vi "Host Input to FPGA_5772_Sine.vi"() -> ()   [LabVIEW 2011]
panel:
  in  "millisecond multiple":u32=20
  out "Trig Offset":u8
  out "16bit integer":i16[](array[numeric])
  out "Init Data":i16[](array[numeric])
  in  "Marker Position":u32
  in  "Frequency":dbl=10000000.0 format="%#_p"
  in  "signal type":T1(ring)
  in  "stop":bool
  out "Data Generated":cluster{"Data":i16, i16}(graph)
  in  "sampling info":cluster{"Fs":dbl, "#s":dbl}={"Fs"=250000000.0, "#s"=100.0} {"Fs" format="%#_p"}
  # "You cannot change waveform type on the fly"
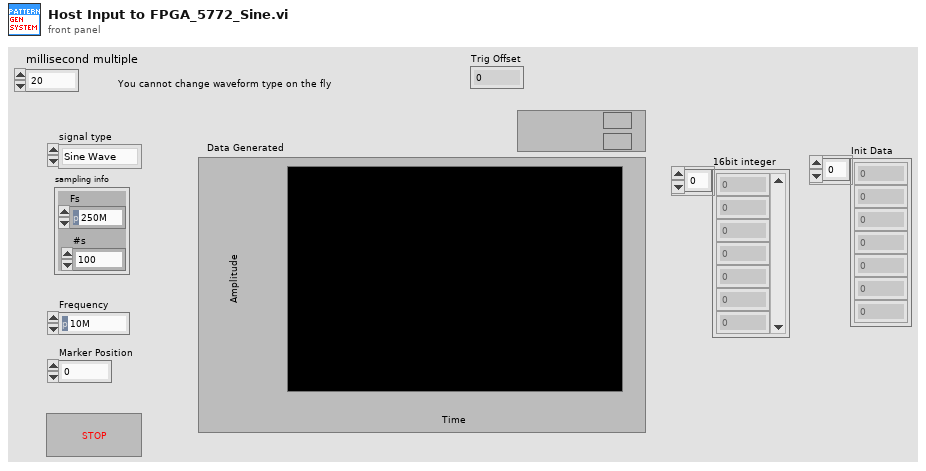
[diagram p1: front panel]
types:
  T1 = enum16{"Sine Wave", "Triangle Wave", "Square Wave", "Sawtooth Wave"}
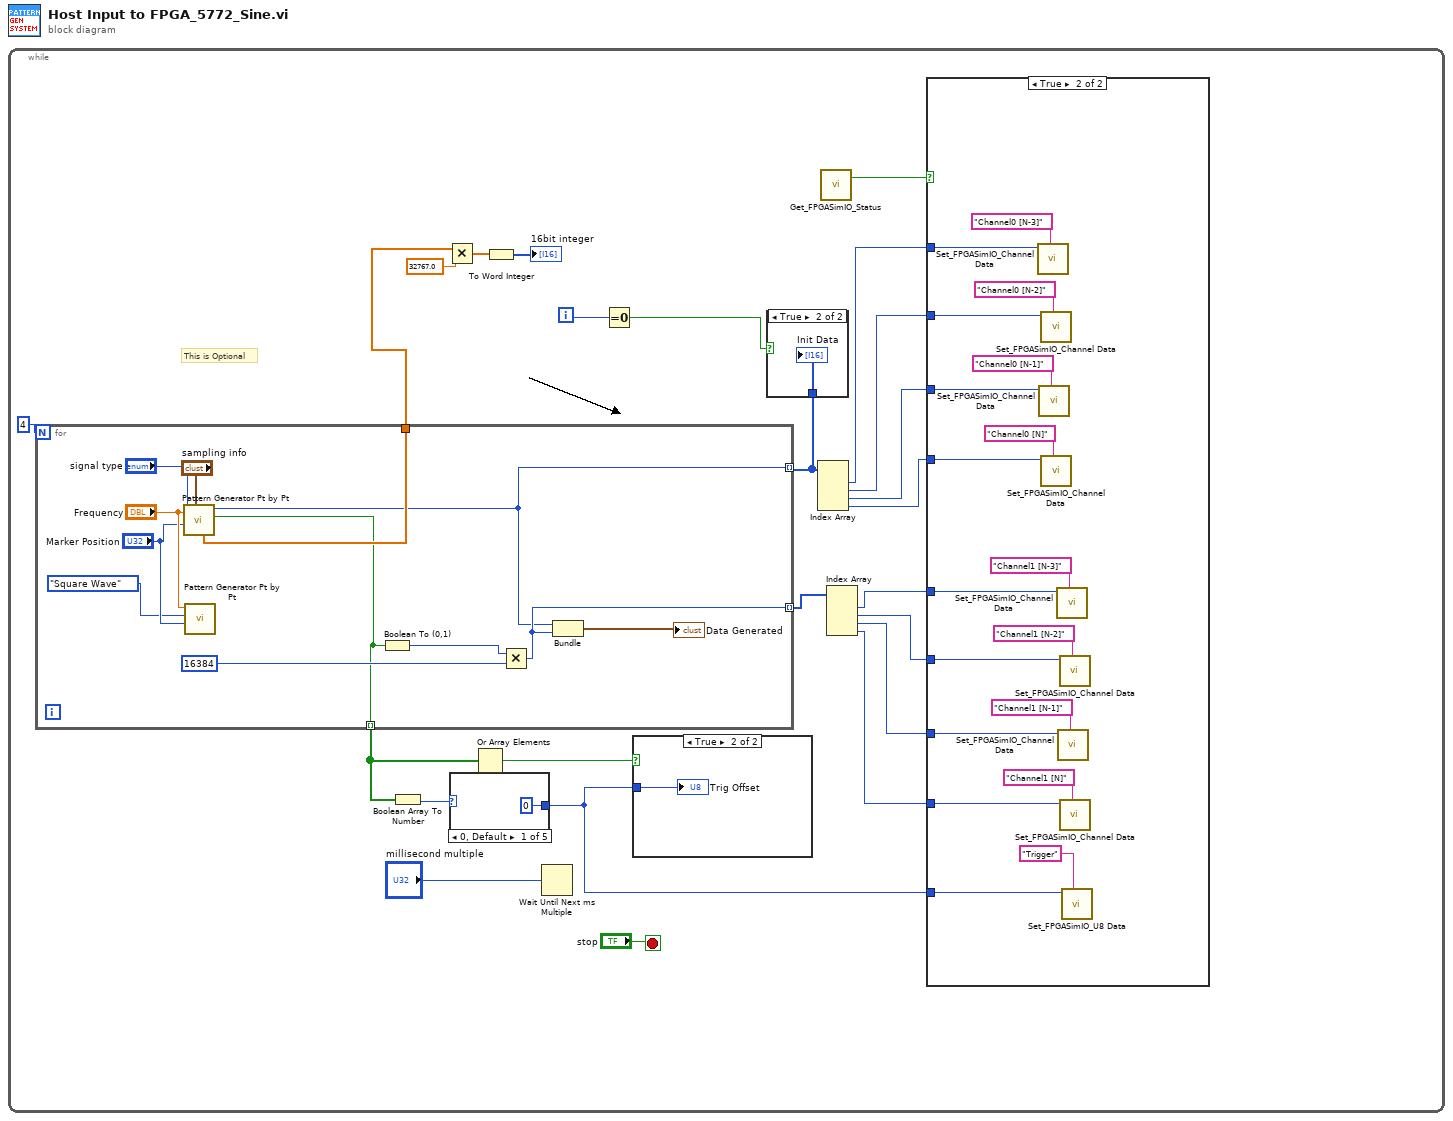
[diagram p0: block diagram]
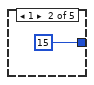
[diagram p2: hidden frame]
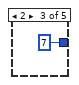
[diagram p3: hidden frame]
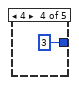
[diagram p4: hidden frame]
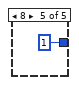
[diagram p5: hidden frame]
diagram:
  n1 = while {
    i -> [w11]
    stop <- "stop" stop-if-true
    # "This is Optional"
    n2 = for {
      N: 4 -> [_]
      tunnel: [w32] -> w12 mode=indexing
      tunnel: [w33] -> w5 mode=indexing
      tunnel: [w35] -> w1 mode=indexing
      tunnel: [w34] -> w7
      n3 = call <userlib>:"Pattern Generator Pt by Pt.vi"("sampling info"="sampling info", "Marker Position"="Marker Position", "signal type"="signal type", "Frequency"="Frequency") -> ("Marker"=w33:bool, "Data"=w32:i16, "Wfm"=w34:dbl[])  [unwired: 4 in, 1 out]
      n4 = call <userlib>:"Pattern Generator Pt by Pt.vi"("Marker Position"="Marker Position", "signal type"=T1."Square Wave", "Frequency"="Frequency") -> ()  [unwired: 5 in, 4 out]
      n5 = Boolean To (0,1)(Boolean=w33) -> (0, 1=w41:i16)
      n6 = Multiply(x=w41, y=i16 16384) -> (x*y=w35:i16)
      n7 = Bundle("Data"=w32, w35) -> (→"Data Generated":cluster{"Data":i16, i16})  [unwired: 1 in]
    }
    n8 = Boolean Array To Number(Boolean array=w5) -> (number=w3:u8)
    n9 = Multiply(x=w7, y=32767.0) -> (x*y=w8:dbl[])
    n10 = case shown="0, Default" w3 {
      tunnel: [u8 0 ("millisecond multiple") u8 15 ("millisecond multiple") u8 7 ("millisecond multiple") u8 3 ("millisecond multiple") u8 1 ("millisecond multiple")] -> w2
      frame 0, Default {
      }
      frame 1 {
      }
      frame 2 {
      }
      frame 4 {
      }
      frame 8 {
      }
    }
    n11 = Or Array Elements(Boolean array=w5) -> (logical OR=w4:bool)
    n12 = To Word Integer(number=w8) -> (16bit integer=→"16bit integer":i16[])
    n13 = Wait Until Next ms Multiple(millisecond multiple="millisecond multiple") -> ()  [unwired: 1 out]
    n14 = Equal To 0?(x=w11) -> (x = 0?=w10:bool)
    n15 = case shown="True" w4 {
      tunnel: w2 -> [_ w30]
      frame False {
      }
      frame True {
        "Trig Offset" <- w30
      }
    }
    n16 = case shown="True" w10 {
      tunnel: w12 -> [_ w31]
      frame False {
      }
      frame True {
        "Init Data" <- w31
      }
    }
    n17 = Index Array(array=w12) -> (element #1=w20:i16, element #2=w19:i16, element #3=w18:i16, element #4=w17:i16)  [unwired: 4 in]
    n18 = call <userlib>:"Get_FPGASimIO_Status.vi"() -> ("Sim IO FPGA Status"=w22:bool)  [unwired: 10 in, 1 out]
    n19 = Index Array(array=w1) -> (element #1=w16:i16, element #2=w15:i16, element #3=w14:i16, element #4=w13:i16)  [unwired: 4 in]
    n20 = case shown="True" w22 {
      tunnel: w20 -> [_ w60]
      tunnel: w19 -> [_ w59]
      tunnel: w18 -> [_ w58]
      tunnel: w17 -> [_ w54]
      tunnel: w16 -> [_ w49]
      tunnel: w15 -> [_ w48]
      tunnel: w14 -> [_ w47]
      tunnel: w13 -> [_ w46]
      tunnel: w2 -> [_ w45]
      frame False {
      }
      frame True {
        n21 = call <userlib>:"Set_FPGASimIO_Channel Data.vi"("Channel Name"="Channel0 [N-3]" ("IO Node Name"), "Data"=w60) -> ()  [unwired: 9 in, 1 out]
        n22 = call <userlib>:"Set_FPGASimIO_Channel Data.vi"("Channel Name"="Channel0 [N-1]" ("IO Node Name"), "Data"=w58) -> ()  [unwired: 9 in, 1 out]
        n23 = call <userlib>:"Set_FPGASimIO_Channel Data.vi"("Channel Name"="Channel0 [N-2]" ("IO Node Name"), "Data"=w59) -> ()  [unwired: 9 in, 1 out]
        n24 = call <userlib>:"Set_FPGASimIO_Channel Data.vi"("Channel Name"="Channel0 [N]" ("IO Node Name"), "Data"=w54) -> ()  [unwired: 9 in, 1 out]
        n25 = call <userlib>:"Set_FPGASimIO_Channel Data.vi"("Channel Name"="Channel1 [N-3]" ("IO Node Name"), "Data"=w49) -> ()  [unwired: 9 in, 1 out]
        n26 = call <userlib>:"Set_FPGASimIO_Channel Data.vi"("Channel Name"="Channel1 [N-1]" ("IO Node Name"), "Data"=w47) -> ()  [unwired: 9 in, 1 out]
        n27 = call <userlib>:"Set_FPGASimIO_Channel Data.vi"("Channel Name"="Channel1 [N-2]" ("IO Node Name"), "Data"=w48) -> ()  [unwired: 9 in, 1 out]
        n28 = call <userlib>:"Set_FPGASimIO_Channel Data.vi"("Channel Name"="Channel1 [N]" ("IO Node Name"), "Data"=w46) -> ()  [unwired: 9 in, 1 out]
        n29 = call <userlib>:"Set_FPGASimIO_U8 Data.vi"("Channel Name"="Trigger", "Data"=w45) -> ()  [unwired: 9 in, 1 out]
      }
    }
  }
